vi "set all (子VI).vi"(4 "Mode(ppms,mpms磁)":i32, 5 "Instrument":T1={"335 Resource"="GPIB0::24::INSTR", "Input (0:A)"=0, "Instrument Type"=enum."PPMS-Rotate", "quantum design"=refnum, "Heater Output (1:1)"=1, "semaphore"=refnum, "TCP master instance"=refnum, "335 Status"=refnum, "M24C Resource"="GPIB0::24::INSTR", "4G supply"="GPIB0::24::INSTR", "Temp Status 24C"=refnum, "Temp"=refnum, "9T信号"=refnum, "limit"={"Field limit"=0.0, "Field rate limit"=0.0, "Temp limit"=0.0, "Temp low limit"=0.0, "Temp rate limit "=0.0}, "4g supply status"=refnum, "vi路径"="", "325 Resource "="GPIB0::24::INSTR", "Input (0:A) 325"=0, "Input (1;B)"=1, "in-plane"="", "out-plane"="", "in-plane"=FALSE, "out-plane"=FALSE, "in plane 信号"=refnum, "pzt volt"=refnum, "Aborting"=refnum, "数据文件"=refnum, "warning"=refnum, "750 visa"="", "750 rotate"="", "335 Status 2"=refnum} {"Input (1;B)" items=["A", "B"]; "Input (0:A) 325" items=["A", "B"]; "Input (0:A)" items=["A", "B"]; "Heater Output (1:1)" items=["1"=1, "2"=2]}, 6 "Approach(ppms, mpms)":i32, 7 "轴向(转角)":enum16{"in plane", "out plane"}(ring), 8 "error in":errorcluster caption="error in (no error)", 9 "Rate/speed":dbl, 10 "Target":dbl, 11 "类型":T5) -> (0 "错误输出":errorcluster)   [LabVIEW 2019, in "User lib.lvlib"]
uses:
  User lib.lvlib
  ctl/set type.ctl
  ctl/Instrument.ctl
  <vilib>/NI/Modbus Library/API/Master/Modbus Master.lvclass
  ctl/Instrument Type.ctl
  lib/QDInstrument.dll
  ctl/335 state.ctl
  ctl/limit.ctl
  ctl/9T mag field stauts.ctl
  ctl/warning.ctl
  SubVI.lvlib
  9T cmag.lvlib
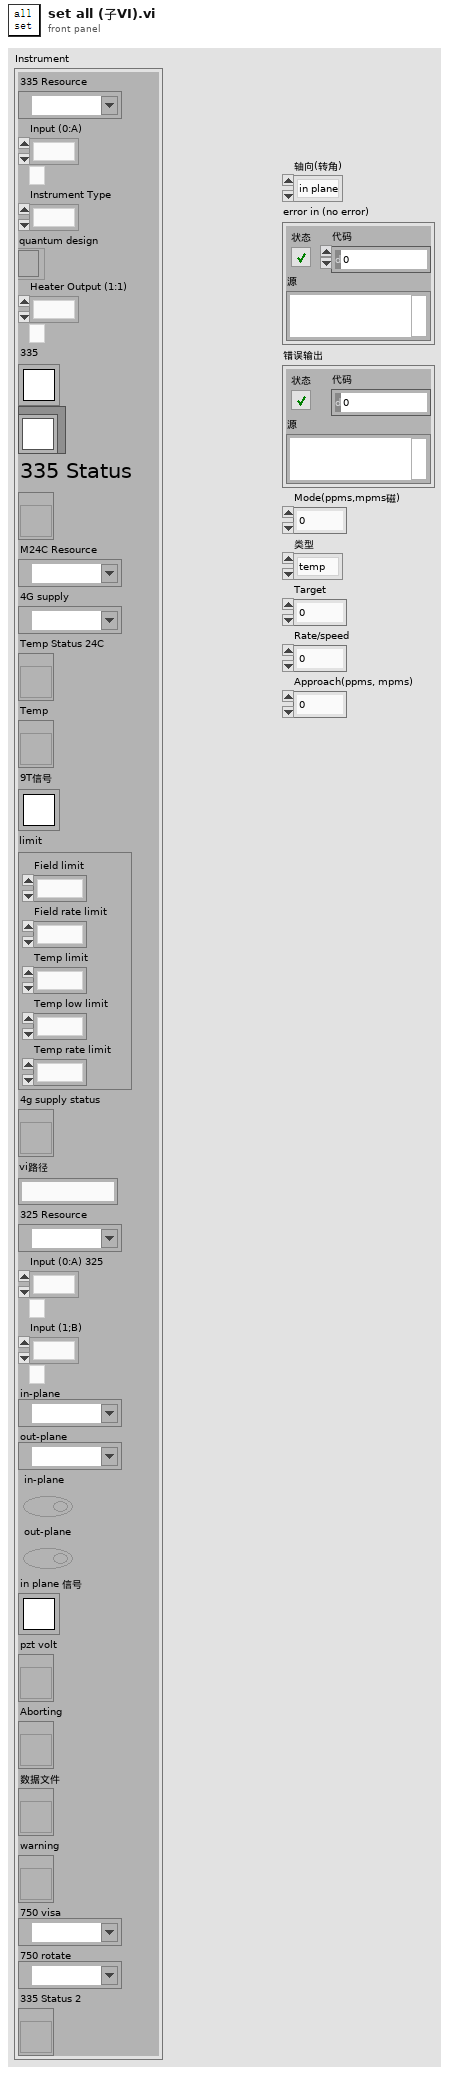
[diagram p1: front panel]
types:
  T1 = typedef "Instrument.ctl" = cluster{"335 Resource":refnum<visa-resource-name>, "Input (0:A)":u16, "Instrument Type":T2, "quantum design":refnum<k24>, "Heater Output (1:1)":u16, "semaphore":T3, "TCP master instance":refnum<class "Modbus Master.lvclass">, "335 Status":refnum<vi>, "M24C Resource":refnum<visa-resource-name>, "4G supply":refnum<visa-resource-name>, "Temp Status 24C":refnum<vi>, "Temp":refnum<vi>, "9T信号":T3, "limit":T4, "4g supply status":refnum<vi>, "vi路径":string, "325 Resource ":refnum<visa-resource-name>, "Input (0:A) 325":u16, "Input (1;B)":u16, "in-plane":refnum<visa-resource-name>, "out-plane":refnum<visa-resource-name>, "in-plane":bool, "out-plane":bool, "in plane 信号":T3, "pzt volt":refnum<vi>, "Aborting":refnum<vi>, "数据文件":refnum<vi>, "warning":refnum<vi>, "750 visa":refnum<visa-resource-name>, "750 rotate":refnum<visa-resource-name>, "335 Status 2":refnum<vi>}
  T2 = typedef "Instrument Type.ctl" = enum16{"PPMS", "VersaLab", "DynaCool", "SVSM", "PPMS-Rotate", "Lakeshore335", "lengtou2", "9T mag", "9T cmag rotate", "test"}
  T3 = typedef "Semaphore RefNum" = refnum<k1>
  T4 = typedef "limit.ctl" = cluster{"Field limit":dbl, "Field rate limit":dbl, "Temp limit":dbl, "Temp low limit":dbl, "Temp rate limit ":dbl}
  T5 = typedef "set type.ctl" = enum16{"temp", "field", "position", "gating"}
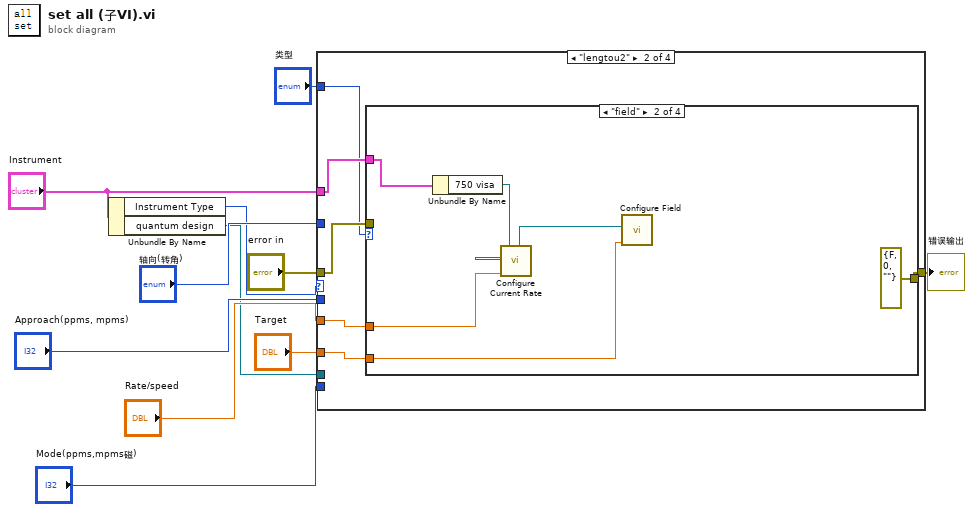
[diagram p0: block diagram]
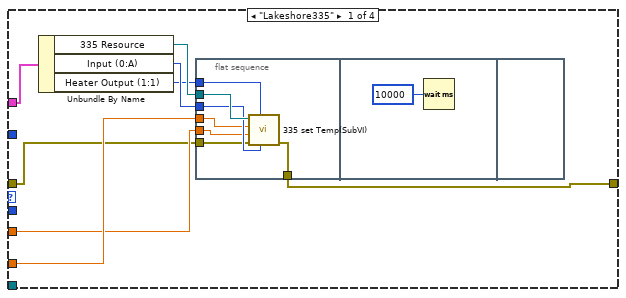
[diagram p2: hidden frame]
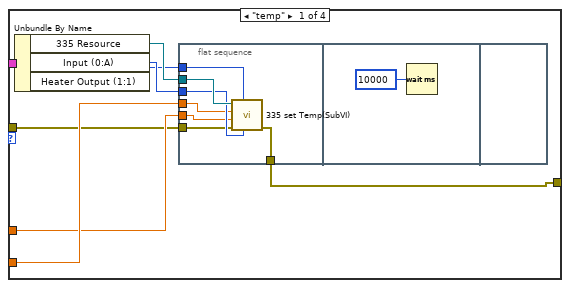
[diagram p3: hidden frame]
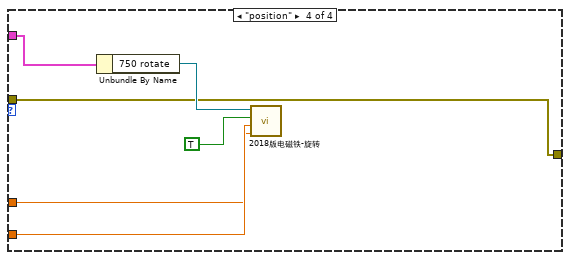
[diagram p5: hidden frame]
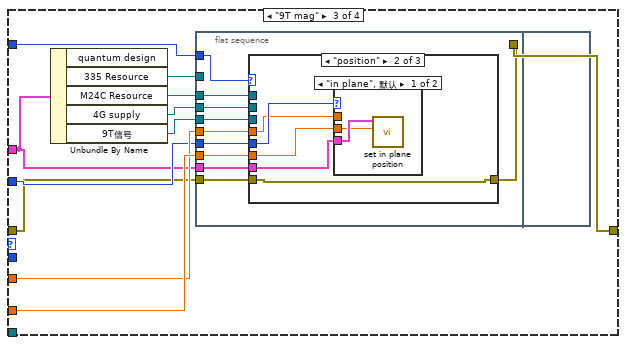
[diagram p6: hidden frame]
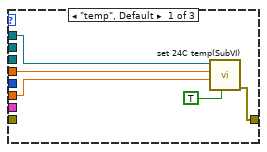
[diagram p7: hidden frame]
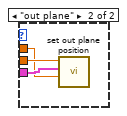
[diagram p8: hidden frame]
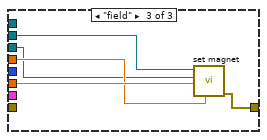
[diagram p9: hidden frame]
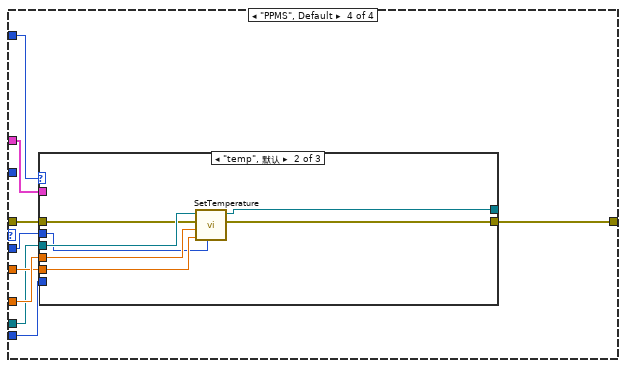
[diagram p10: hidden frame]
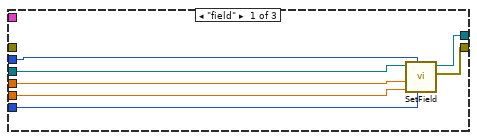
[diagram p11: hidden frame]
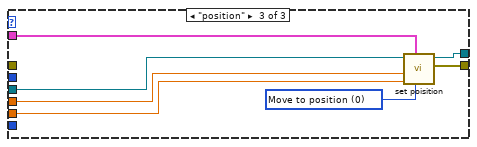
[diagram p12: hidden frame]
diagram:
  n1 = Unbundle By Name("Instrument") -> ("Instrument Type"=w3:T2, "quantum design"=w2:refnum<k24>)
  n2 = case shown="\"lengtou2\"" w3 {
    tunnel: "Target" -> [w16 w33 w72 w112]
    tunnel: "Mode(ppms,mpms磁)" -> [_ _ _ w111]
    tunnel: "Approach(ppms, mpms)" -> [_ _ _ w110]
    tunnel: "Rate/speed" -> [w15 w32 w71 w109]
    tunnel: w2 -> [_ _ _ w108]
    tunnel: [w14 w31 w70 w107] -> w9
    tunnel: "类型" -> [_ w28 w68 w106]
    tunnel: "Instrument" -> [w13 w30 w63 w105]
    tunnel: "轴向(转角)" -> [_ _ w65 _]
    tunnel: "error in" -> [w12 w29 w64 w104]
    frame "Lakeshore335" {
      n3 = Unbundle By Name(w13) -> ("335 Resource"=w19:refnum<visa-resource-name>, "Input (0:A)"=w18:u16, "Heater Output (1:1)"=w17:u16)
      n4 = flat-sequence {
        tunnel: w19 -> [w26]
        tunnel: w18 -> [w25]
        tunnel: w17 -> [w24]
        tunnel: w16 -> [w23]
        tunnel: w15 -> [w22]
        tunnel: [w21] -> w14
        tunnel: w12 -> [w20]
        frame #0 {
          n5 = call "335 set Temp(SubVI).vi"("Input (0:A)"=w25, "Output (1:1)"=w24, "error in (no error)"=w20, "Rate"=w22, "Temperature"=w23, "VISA Refnum in"=w26) -> ("error out"=w21:errorcluster)  [unwired: 4 in, 1 out]
        }
        frame #1 {
          n6 = Wait (ms)(milliseconds to wait=u32 10000 ("等待时间（毫秒）")) -> ()  [unwired: 1 out]
        }
        frame #2 {
        }
      }
    }
    frame "lengtou2" {
      n7 = case shown="\"field\"" w28 {
        tunnel: w33 -> [w38 w53 _ w60]
        tunnel: w32 -> [w37 w52 _ w59]
        tunnel: [w36 errorcluster {"status"=FALSE, "code"=0, "source"=""} ("error out") w56 w57] -> w31
        tunnel: w30 -> [w35 w54 _ w62]
        tunnel: w29 -> [w34 _ w56 w57]
        frame "temp" {
          n8 = Unbundle By Name(w35) -> ("335 Resource"=w41:refnum<visa-resource-name>, "Input (0:A)"=w40:u16, "Heater Output (1:1)"=w39:u16)
          n9 = flat-sequence {
            tunnel: w41 -> [w48]
            tunnel: w40 -> [w47]
            tunnel: w39 -> [w46]
            tunnel: w38 -> [w45]
            tunnel: w37 -> [w44]
            tunnel: [w43] -> w36
            tunnel: w34 -> [w42]
            frame #0 {
              n10 = call "335 set Temp(SubVI).vi"("Input (0:A)"=w47, "Output (1:1)"=w46, "error in (no error)"=w42, "Rate"=w44, "Temperature"=w45, "VISA Refnum in"=w48) -> ("error out"=w43:errorcluster)  [unwired: 4 in, 1 out]
            }
            frame #1 {
              n11 = Wait (ms)(milliseconds to wait=u32 10000 ("等待时间（毫秒）")) -> ()  [unwired: 1 out]
            }
            frame #2 {
            }
          }
        }
        frame "field" {
          n12 = Unbundle By Name(w54) -> ("750 visa"=w51:refnum<visa-resource-name>)
          n13 = call "Configure Current Rate.vi"("Current Rate（A/S）"=w52, "VISA resource name"=w51) -> ("VISA resource name out"=w50:refnum<visa-resource-name>)  [unwired: 8 in, 1 out]
          n14 = call "Configure Field.vi"("Field（Gs）"=w53, "VISA resource name"=w50) -> ()  [unwired: 8 in, 2 out]
        }
        frame "gating", Default {
        }
        frame "position" {
          n15 = Unbundle By Name(w62) -> ("750 rotate"=w61:refnum<visa-resource-name>)
          n16 = call "2018版电磁铁-旋转.vi"("速度选择"=w59, "设定角度"=w60, "方向选择"=TRUE, "VISA资源名称"=w61) -> ()  [unwired: 8 in]
        }
      }
    }
    frame "9T mag" {
      n17 = Unbundle By Name(w63) -> ("335 Resource"=w73:refnum<visa-resource-name>, "M24C Resource"=w69:refnum<visa-resource-name>, "4G supply"=w67:refnum<visa-resource-name>, "9T信号"=w66:T3)  [unwired: 1 out]
      n18 = flat-sequence {
        tunnel: w73 -> [_]
        tunnel: w72 -> [w81]
        tunnel: w71 -> [w82]
        tunnel: [w80] -> w70
        tunnel: w69 -> [w83]
        tunnel: w68 -> [w79]
        tunnel: w67 -> [w78]
        tunnel: w66 -> [w77]
        tunnel: w65 -> [w76]
        tunnel: w63 -> [w75]
        tunnel: w64 -> [w74]
        frame #0 {
          n19 = case shown="\"position\"" w79 {
            tunnel: w83 -> [w88 _ _]
            tunnel: w82 -> [w87 w90 w101]
            tunnel: w81 -> [w86 w91 w102]
            tunnel: [w85 w89 w100] -> w80
            tunnel: w78 -> [_ _ w103]
            tunnel: w77 -> [_ _ w99]
            tunnel: w76 -> [_ w93 _]
            tunnel: w75 -> [_ w92 _]
            tunnel: w74 -> [_ w89 _]
            frame "temp", Default {
              n20 = call "set 24C temp(SubVI).vi"("Control"=TRUE, "Temperature"=w86, "Rate"=w87, "VISA引用句柄输入"=w88) -> ("ErrorOut"=w85:errorcluster)  [unwired: 7 in]
            }
            frame "position" {
              n21 = case shown="\"in plane\", 默认" w93 {
                tunnel: w92 -> [w95 w98]
                tunnel: w91 -> [w94 w97]
                tunnel: w90 -> [_ w96]
                frame "in plane", Default {
                  n22 = call "set in plane position.vi"("Value"=w94, "Instrument"=w95) -> ()  [unwired: 10 in]
                }
                frame "out plane" {
                  n23 = call "set out plane position.vi"("Speed"=w96, "Instrument"=w98, "Value"=w97) -> ()  [unwired: 9 in]
                }
              }
            }
            frame "field" {
              n24 = call "set magnet.vi"("Rate(Oe/s)"=w101, "Magnet field(Oe)"=w102, "semaphore"=w99, "VISA Resource Name"=w103) -> ("error out"=w100:errorcluster)  [unwired: 5 in, 2 out]
            }
          }
        }
        frame #1 {
        }
      }
    }
    frame "PPMS", Default {
      n25 = case shown="\"temp\", 默认" w106 {
        tunnel: w112 -> [w119 w125 w130]
        tunnel: w111 -> [w118 _ _]
        tunnel: w110 -> [w117 w123 _]
        tunnel: w109 -> [w116 w124 w129]
        tunnel: w108 -> [w115 w126 w133]
        tunnel: [w114 w122 w132] -> _
        tunnel: [w113 w121 w131] -> w107
        tunnel: w105 -> [_ _ w128]
        tunnel: w104 -> [_ w120 _]
        frame "field" {
          n26 = call "SetField.vi"("Mode"=w118, "Approach"=w117, "Rate"=w116, "Field"=w119, "Instrument Ref In"=w115) -> ("error out"=w113:errorcluster, "Instrument Ref Out"=w114:refnum<k24>)  [unwired: 2 in, 1 out]
        }
        frame "temp", Default {
          n27 = call "SetTemperature.vi"("Approach"=w123, "Rate"=w124, "Temperature"=w125, "error in (no error)"=w120, "Instrument Ref In"=w126) -> ("error out"=w121:errorcluster, "Instrument Ref Out"=w122:refnum<k24>)  [unwired: 2 in, 1 out]
        }
        frame "position" {
          w127 = u16 0 items=["Move to position", "Move to limit", "Redefine current position"] ("Mode")
          n28 = call "set poisition.vi"("Mode"=w127, "Instrument"=w128, "Slow down code\ndefault = 0"=w129, "Position (deg)"=w130, "Instrument Ref In"=w133) -> ("error out"=w131:errorcluster, "Instrument Ref Out"=w132:refnum<k24>)  [unwired: 3 in]
        }
      }
    }
  }
  "错误输出" <- w9
